vi "ReadData.vi"(11 "scope params":T1={"scope mode"=enum."Stopped", "ticker"=refnum, "samples per simulated"=0, "FPGA ref"=refnum, "P2P params"={"instrument handle"="", "stream session"=refnum, "scale"={"offset"=0.0, "gain"=0.0, "reserved 1"=0.0, "reserved 2"=0.0}, "actual sample rate"=10000000.0, "Trigger"=enum."PFI 0", "SCOPE Resource"="Dev1", "input impedance"=0}, "data mode"=enum."Real IO"} {"P2P params"."input impedance" items=["1 mega ohm"=0, "50 ohms"=2]; "P2P params"."actual sample rate" format="%.2p"}) -> (1 "Num elements":i32, 2 "data":i16[][](array[numeric]), 3 "scope params out":T1={"scope mode"=enum."Stopped", "ticker"=refnum, "samples per simulated"=0, "FPGA ref"=refnum, "P2P params"={"instrument handle"="", "stream session"=refnum, "scale"={"offset"=0.0, "gain"=0.0, "reserved 1"=0.0, "reserved 2"=0.0}, "actual sample rate"=10000000.0, "Trigger"=enum."PFI 0", "SCOPE Resource"="Dev1", "input impedance"=0}, "data mode"=enum."Real IO"} {"P2P params"."input impedance" items=["1 mega ohm"=0, "50 ohms"=2]; "P2P params"."actual sample rate" format="%.2p"})   [LabVIEW 2013]
uses:
  controls/scope_params.ctl
  Utilities/Ticker/Ticker.lvclass
  controls/ScopeMode.ctl
  Config/FPGAref.ctl
  P2P streaming/P2P params.ctl
  P2P streaming/trigger_source.ctl
  FPGA/DataMode.ctl
  <vilib>/rvi/interface/common/niFpgaWaitOnOcc.vi
  <vilib>/Utility/error.llb/Error Cluster From Error Code.vi
  <vilib>/rvi/errors/niLvFpgaAdjustHostInterfaceError.vi
  <vilib>/rvi/interface/nirviMethod/nirviMethod.xnode
  <vilib>/rvi/interface/nirviReadWriteControl/nirviReadWriteControl.xnode
  NiFpgaLv.dll
  <vilib>/rvi/interface/Simulation/niFpgaSimulationCallBeginRW.vi
  <vilib>/FPGAPlugInAG/Dynamic/niLvFpga_ReadFifo_Dynamic.vi
  <vilib>/rvi/errors/niLvFpgaMergeErrorWithErrorCode.vi
panel:
  out "Data":u64[](array[numeric])
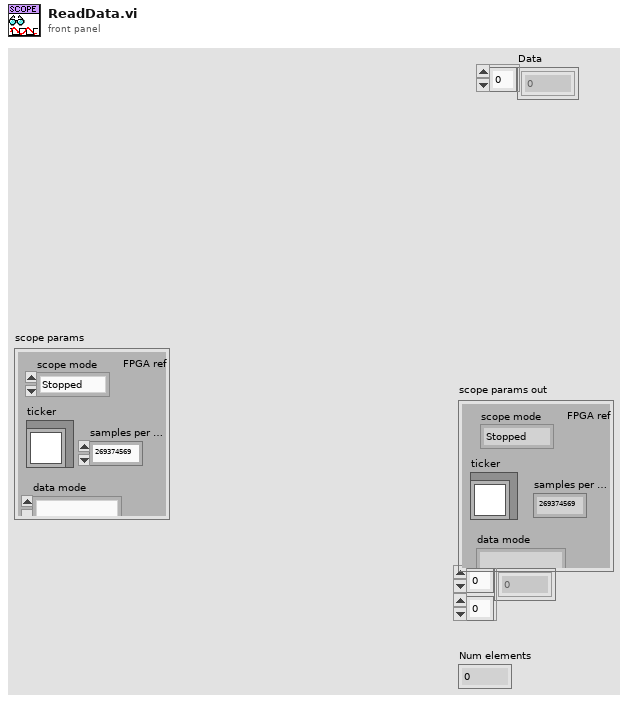
[diagram p1: front panel]
types:
  T1 = typedef "scope_params.ctl" = cluster{"scope mode":T2, "ticker":refnum<class "Ticker.lvclass">, "samples per simulated":u32, "FPGA ref":T3, "P2P params":T4, "data mode":T6}
  T2 = typedef "ScopeMode.ctl" = enum16{"Stopped", "Single", "Running"}
  T3 = typedef "FPGAref.ctl" = refnum<k20>
  T4 = typedef "P2P params.ctl" = cluster{"instrument handle":refnum<k15>, "stream session":refnum<k20>, "scale":cluster{"offset":dbl, "gain":dbl, "reserved 1":dbl, "reserved 2":dbl}, "actual sample rate":dbl, "Trigger":T5, "SCOPE Resource":refnum<k15>, "input impedance":u32}
  T5 = typedef "trigger_source.ctl" = enum16{"PFI 0", "PFI 1", "Software"}
  T6 = typedef "DataMode.ctl" = enum16{"Real IO", "Simulated"}
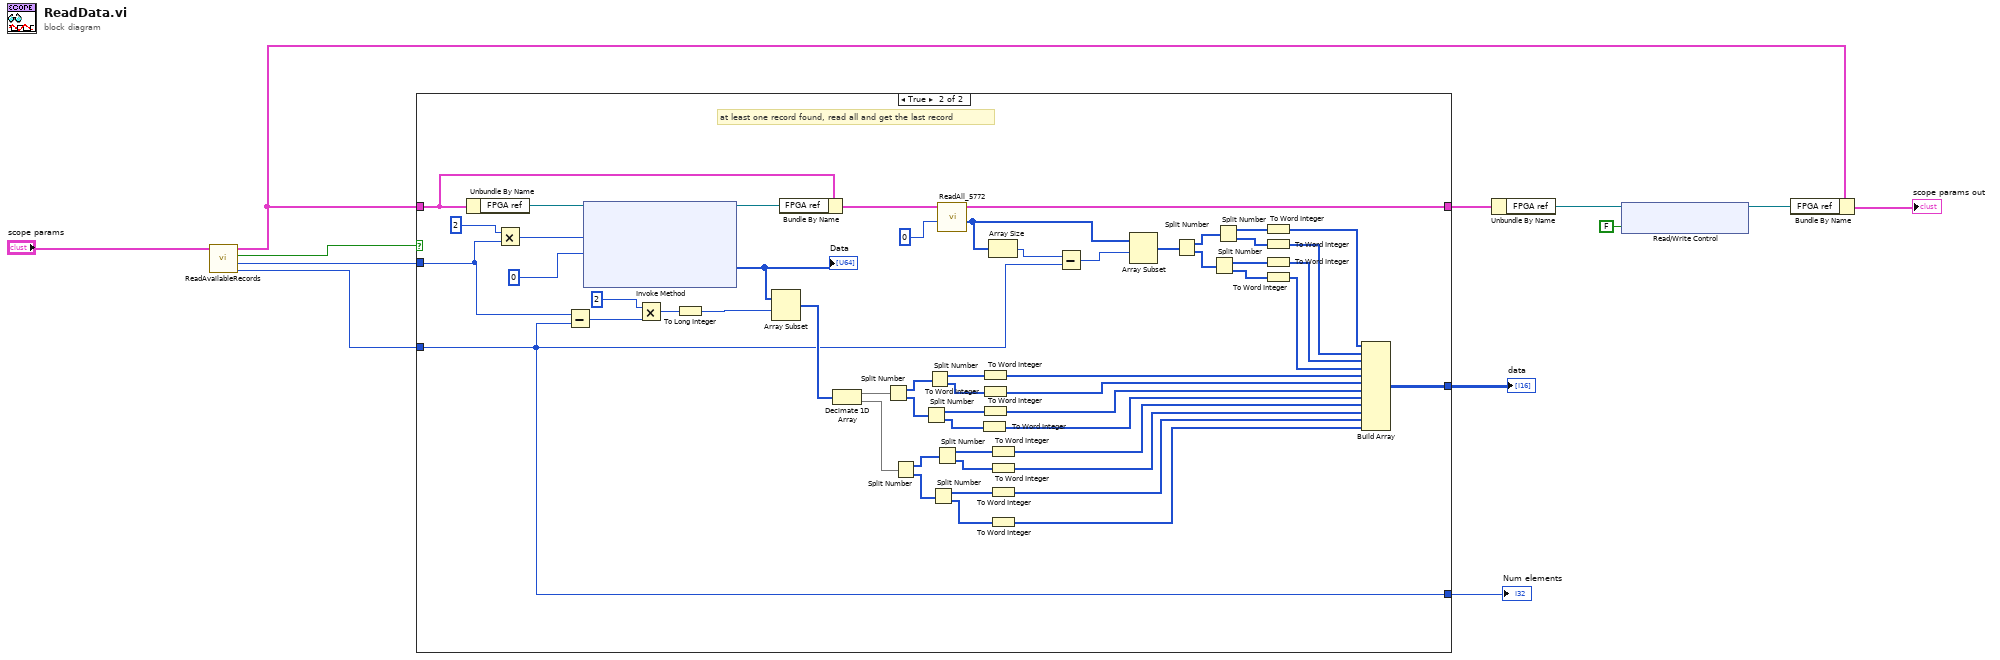
[diagram p0: block diagram]
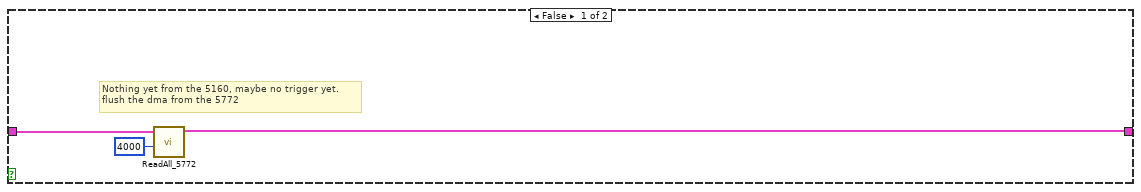
[diagram p2: hidden frame]
diagram:
  n1 = call "ReadAvailableRecords.vi"("scope params"="scope params") -> ("last record size"=w4:u32, "#elements"=w5:u32, "record available"=w6:bool, "scope params out"=w3:T1)  [unwired: 7 in]
  n2 = case shown="True" w6 {
    tunnel: [_ w26] -> w12
    tunnel: [_ w23] -> w11
    tunnel: w5 -> [_ w20]
    tunnel: w4 -> [_ w23]
    tunnel: w3 -> [w15 w43]
    tunnel: [w14 w39] -> w2
    frame False {
      # "Nothing yet from the 5160, maybe no trigger yet.\nflush the dma from the 5772"
      n3 = call "ReadAll_5772.vi"("# elements to keep in DMA"=u32 4000, "scope params"=w15) -> ("scope params"=w14:T1)  [unwired: 8 in, 1 out]
    }
    frame True {
      # "at least one record found, read all and get the last record"
      n4 = Unbundle By Name(w43) -> ("FPGA ref"=w44:T3)
      n5 = Multiply(x=u32 2, y=w20) -> (x*y=w19:u32)
      n6 = Subtract(x=w20, y=w23) -> (x-y=w17:u32)
      n7 = xnode "Invoke Method"("FPGA VI Reference In"=w44, "Number of Elements"=w19, "Timeout (ms)"=0) -> ("FPGA VI Reference Out"=w42:T3, "Data"=w46:u64[])  [unwired: 1 in, 2 out]
      "Data" <- w46
      n8 = Multiply(x=u32 2, y=w17) -> (x*y=w16:u32)
      n9 = To Long Integer(number=w16) -> (32bit integer=w38:i32)
      n10 = Array Subset(array=w46, index=w38) -> (w47:u64[])  [unwired: 1 in]
      n11 = Bundle By Name(cluster=w43, "FPGA ref"=w42) -> (w41:T1)
      n12 = Decimate 1D Array(w47) -> (w63:u64[], w52:u64[])
      n13 = Split Number(x=w63) -> (hi(x)=w65:u32[], lo(x)=w69:u32[])
      n14 = Split Number(x=w52) -> (hi(x)=w57:u32[], lo(x)=w53:u32[])
      n15 = Split Number(x=w69) -> (hi(x)=w67:u16[], lo(x)=w66:u16[])
      n16 = Split Number(x=w65) -> (hi(x)=w64:u16[], lo(x)=w68:u16[])
      n17 = Split Number(x=w53) -> (hi(x)=w55:u16[], lo(x)=w56:u16[])
      n18 = Split Number(x=w57) -> (hi(x)=w58:u16[], lo(x)=w54:u16[])
      n19 = call "ReadAll_5772.vi"("# elements to keep in DMA"=u32 0, "scope params"=w41) -> ("Data"=w25:u64[], "scope params"=w39:T1)  [unwired: 8 in]
      n20 = To Word Integer(number=w66) -> (16bit integer=w59:i16[])
      n21 = To Word Integer(number=w64) -> (16bit integer=w62:i16[])
      n22 = To Word Integer(number=w68) -> (16bit integer=w61:i16[])
      n23 = To Word Integer(number=w67) -> (16bit integer=w60:i16[])
      n24 = Array Size(array=w25) -> (size(s)=w24:i32)
      n25 = To Word Integer(number=w58) -> (16bit integer=w51:i16[])
      n26 = To Word Integer(number=w54) -> (16bit integer=w50:i16[])
      n27 = To Word Integer(number=w55) -> (16bit integer=w49:i16[])
      n28 = To Word Integer(number=w56) -> (16bit integer=w48:i16[])
      n29 = Subtract(x=w24, y=w23) -> (x-y=w22:u32)
      n30 = Array Subset(array=w25, index=w22) -> (w31:u64[])  [unwired: 1 in]
      n31 = Split Number(x=w31) -> (hi(x)=w37:u32[], lo(x)=w36:u32[])
      n32 = Split Number(x=w36) -> (hi(x)=w34:u16[], lo(x)=w33:u16[])
      n33 = Split Number(x=w37) -> (hi(x)=w32:u16[], lo(x)=w35:u16[])
      n34 = To Word Integer(number=w32) -> (16bit integer=w27:i16[])
      n35 = To Word Integer(number=w35) -> (16bit integer=w28:i16[])
      n36 = To Word Integer(number=w34) -> (16bit integer=w29:i16[])
      n37 = To Word Integer(number=w33) -> (16bit integer=w30:i16[])
      n38 = Build Array(w27, w28, w29, w30, w62, w61, w60, w59, w51, w50, w49, w48) -> (w26:i16[][])
    }
  }
  "data" <- w12
  "Num elements" <- w11
  n39 = Unbundle By Name(w2) -> ("FPGA ref"=w1:T3)
  n40 = xnode "Read/Write Control"("FPGA VI Reference In"=w1, "Trigger simulated data"=FALSE) -> ("FPGA VI Reference Out"=w9:T3)  [unwired: 1 in, 1 out]
  n41 = Bundle By Name(cluster=w3, "FPGA ref"=w9) -> (→"scope params out":T1)
